vi "auto left.vi"() -> ()   [LabVIEW 2012, in "Omni2013.lvrbt"]
uses:
  Omni2013.lvrbt
  <vilib>/NXT/Hardware/Plugins/Tetrix 180 deg Servo/Tetrix180ServoAddress.ctl
  <vilib>/NXT/Hardware/Plugins/Tetrix DC Motor/TetrixDCMotorAddress.ctl
  <vilib>/NXT/Block Support/NXT_InputPort.ctl
  <vilib>/NXT/HiTechnic/HiTechnic Controls/HiTechnic Port.ctl
  <vilib>/NXT/Dual Mode Library/Waits/Wait_Num(msec).vi
  <vilib>/NXT/NXTIO Xnodes/NXTIONodeSubVIs/TETRIX IO Move Servos.vi
  <vilib>/NXT/NXTIO Xnodes/NXTIONodeSubVIs/TETRIX IO Move DC Motors.vi
  <vilib>/NXT/HiTechnic/HiTechnic Config/HiTechnic IRSeeker Mode1200Hz.vi
  <vilib>/NXT/Dual Mode Library/Sensors/Sonar_cm.vi
  <vilib>/NXT/Dual Mode Library/Display/drawNumber.vi
  <vilib>/NXT/HiTechnic/HiTechnic Read/HiTechnic IRSeeker Sensor_DC all.vi
  <vilib>/NXT/Dual Mode Library/Sensors/Light_On.vi
  <vilib>/NXT/NXTIO Xnodes/AddressXNode/NXTIOAddress.xnode
  <vilib>/NXT/NXTIO Xnodes/NXTIOXNode/NXTIO.xnode
  <vilib>/NXT/Subs/LVHSConnector.ctl
  <vilib>/NXT/LegoClasses/BrickReference/BrickReference.lvclass
panel:
  in  "Rotation":dbl
  in  "Translation L&R":dbl
  in  "Translation U&D":dbl
  in  "Initial Time":dbl
  out "Enabled":bool
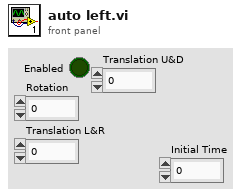
[diagram p1: front panel]
types:
  T1 = typedef "LVHSConnector.ctl" = refnum<class "BrickReference.lvclass">
  T2 = typedef "HiTechnic Port.ctl" = cluster{"Port":T3, "MUX Port":u8}
  T3 = typedef "NXT_InputPort.ctl" = u8
  T4 = typedef "TetrixDCMotorAddress.ctl" = i16
  T5 = cluster{"TetrixDCMotor":T4, "TetrixDCMotor 2":T4}
  T6 = typedef "Tetrix180ServoAddress.ctl" = i16
  T7 = cluster{"Direction (0-9)":i16, "Signal Strength (Array)":u8[]}
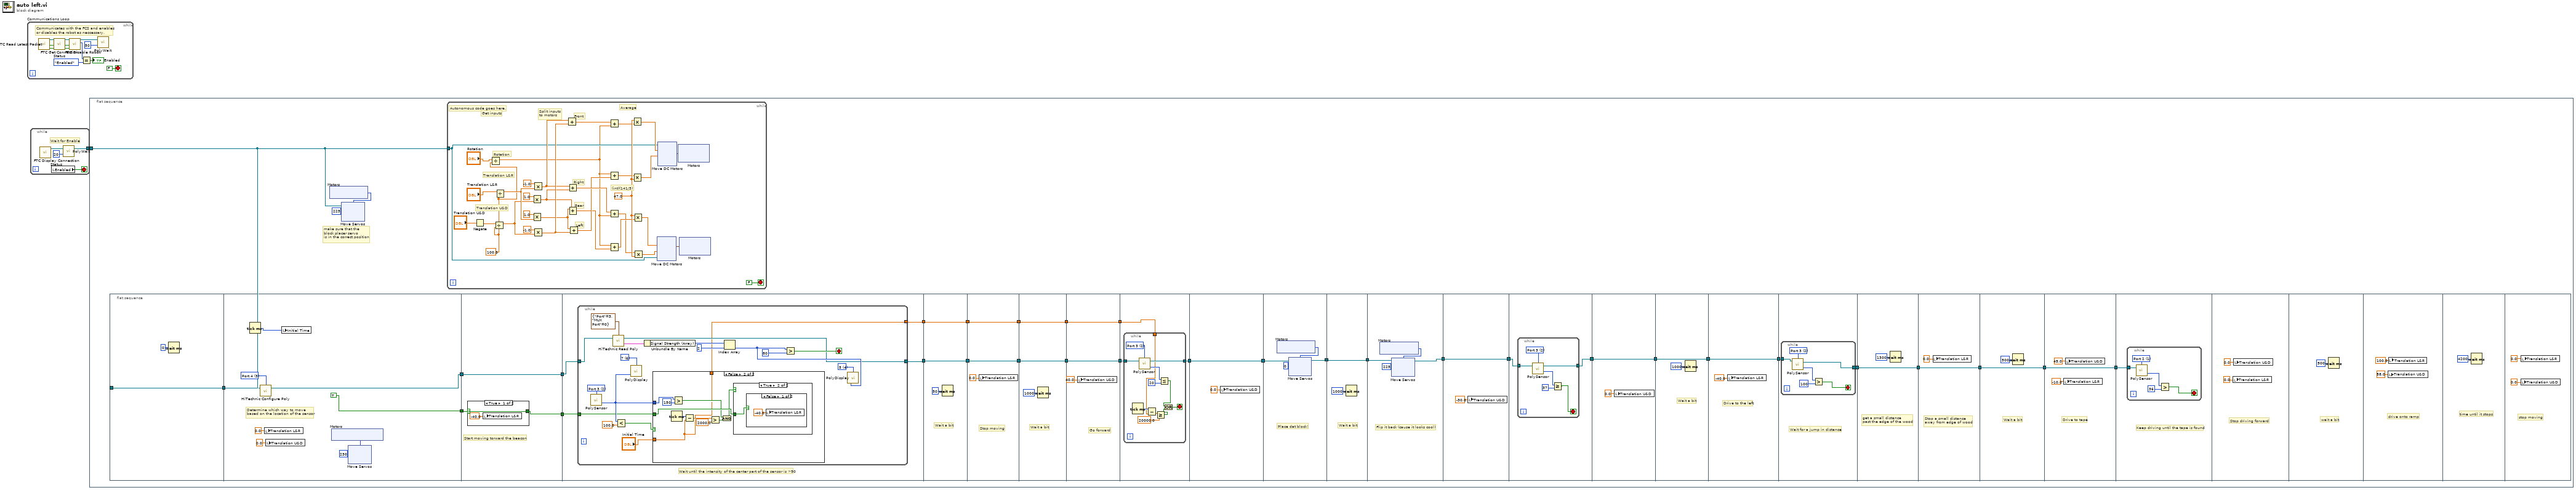
[diagram p0: block diagram]
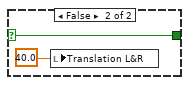
[diagram p2: hidden frame]
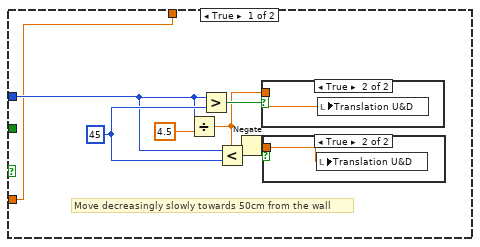
[diagram p3: hidden frame]
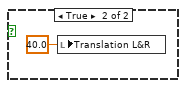
[diagram p7: hidden frame]
diagram:
  n1 = while "Communications Loop" {
    stop <- FALSE stop-if-true
    # "Communicates with the FCS and enables \nor disables the robot as neccessary."
    n2 = call <vilib>:"FTC Read Latest Packet.vi"() -> ("Packet Received?"=w11:bool, "Stopped?"=w10:bool, "NXT"=w13:T1)  [unwired: 6 in, 3 out]
    n3 = call <vilib>:"FTC Get Connection Status.vi"("Packet Received?"=w11, "Stopped?"=w10, "NXT"=w13) -> ("Online?"=w2:bool, "Stopped?"=w3:bool, "NXT"=w12:T1)  [unwired: 5 in]
    n4 = call <vilib>:"FTC Disable Robot.vi"("Online?"=w2, "Stopped?"=w3, "NXT"=w12) -> ("Enabled?"=w6:enum16{"Disabled", "Enabled"}, "NXT"=w8:T1)  [unwired: 3 in]
    n5 = Equal?(x=w6, y=enum16{"Disabled", "Enabled"}."Enabled") -> (x = y?=→"Enabled":bool)
    n6 = call-poly <vilib>:"PolyWait.vi"("Time (100 msec)"=u32 50 ("Time (msec)"), "NXT"=w8) -> ()  [unwired: 2 in, 1 out]
  }
  n7 = while {
    tunnel: [w15] -> w1
    stop <- w16 stop-if-true
    # "Wait for Enable"
    n8 = call <vilib>:"FTC Display Connection Status.vi"() -> ("NXT"=w14:T1)  [unwired: 11 in]
    n9 = local read "Enabled"() -> (w16:bool)
    n10 = call-poly <vilib>:"PolyWait.vi"("Time (100 msec)"=u32 20 ("Time (msec)"), "NXT"=w14) -> ("NXT"=w15:T1)  [unwired: 2 in]
  }
  n11 = flat-sequence {
    tunnel: w1 -> [w48]
    frame #0 {
      # "make sure that the \nblock placer servo \nis in the correct position"
      n12 = flat-sequence {
        tunnel: w48 -> [w60]
        tunnel: [w60] -> w29
        tunnel: [TRUE] -> w31
        tunnel: [w68] -> w30
        tunnel: w29 -> [w64]
        tunnel: [w80] -> w45
        tunnel: w31 -> [w79]
        tunnel: w30 -> [w80]
        tunnel: [w78] -> w39
        tunnel: w45 -> [w88]
        tunnel: [w87] -> w47
        tunnel: w39 -> [w86]
        tunnel: [w85] -> w18
        tunnel: w47 -> [w132]
        tunnel: [w132] -> w46
        tunnel: [w130] -> w19
        tunnel: w18 -> [w130]
        tunnel: [w134] -> w44
        tunnel: w46 -> [w134]
        tunnel: [w133] -> w20
        tunnel: w19 -> [w133]
        tunnel: [w138] -> w40
        tunnel: w44 -> [w138]
        tunnel: [w136] -> w21
        tunnel: w20 -> [w136]
        tunnel: w40 -> [w141]
        tunnel: [w141] -> w43
        tunnel: [w139] -> w22
        tunnel: w21 -> [w139]
        tunnel: w43 -> [w144]
        tunnel: [w143] -> w28
        tunnel: w22 -> [w142]
        tunnel: [w157] -> w27
        tunnel: w28 -> [w157]
        tunnel: w27 -> [w160]
        tunnel: [w159] -> w42
        tunnel: w42 -> [w172]
        tunnel: [w172] -> w41
        tunnel: w41 -> [w174]
        tunnel: [w173] -> w26
        tunnel: w26 -> [w186]
        tunnel: [w186] -> w25
        tunnel: w25 -> [w188]
        tunnel: [w187] -> w24
        tunnel: w24 -> [w196]
        tunnel: [w196] -> w23
        tunnel: [w197] -> w37
        tunnel: w23 -> [w197]
        tunnel: [w199] -> w38
        tunnel: w37 -> [w199]
        tunnel: w38 -> [w202]
        tunnel: [w201] -> w32
        tunnel: [w209] -> w33
        tunnel: w32 -> [w209]
        tunnel: [w211] -> w34
        tunnel: w33 -> [w211]
        tunnel: [w213] -> w35
        tunnel: w34 -> [w213]
        tunnel: [w215] -> w36
        tunnel: w35 -> [w215]
        tunnel: w36 -> [w218]
        frame #0 {
          n13 = Wait (ms)(milliseconds to wait=u32 0) -> ()  [unwired: 1 out]
        }
        frame #1 {
          w67 = T3 3 items=["Port 1", "Port 2", "Port 3", "Port 4"] ("Port")
          # "Determine which way to move \nbased on the location of the sensor"
          n14 = Tick Count (ms)() -> (millisecond timer value=w63:u32)
          n15 = call-poly <vilib>:"HiTechnic Configure Poly.vi"("NXT"=w64, "Port"=w67) -> ("NXT"=w68:T1)  [unwired: 2 in]
          n16 = local write "Translation L&R"(0.0 ("Translation L&R")) -> ()
          n17 = local write "Translation U&D"(0.0 ("Translation U&D")) -> ()
          n18 = local write "Initial Time"(w63) -> ()
          n19 = xnode "Motors"() -> ("Motor"=w62:T6)
          n20 = xnode "Move Servos"("Position 1"=u8 230, "Servos"=w62) -> ()  [unwired: 1 in, 1 out]
        }
        frame #2 {
          # "Start moving torward the beacon"
          n21 = case shown="True" w79 {
            selector: w79 -> [w81 w83]
            tunnel: [w81 w83] -> w78
            frame True {
              n22 = local write "Translation L&R"(-40.0 ("Translation L&R")) -> ()
            }
            frame False {
              n23 = local write "Translation L&R"(40.0 ("Translation L&R")) -> ()
            }
          }
        }
        frame #3 {
          # "Wait until the intensity of the center part of the sensor is >90"
          n24 = while {
            tunnel: w88 -> [w98]
            tunnel: [w96] -> w87
            tunnel: w86 -> [w91]
            tunnel: [w90] -> w85
            stop <- w102 stop-if-true
            w95 = i16 6 items=["1", "2", "3", "4", "5", "6", "7", "8"] ("Line")
            w97 = T3 2 items=["Port 1", "Port 2", "Port 3", "Port 4"] ("Port (Port 4)")
            w101 = i16 4 items=["1", "2", "3", "4", "5", "6", "7", "8"] ("Line")
            n25 = call-poly <vilib>:"PolySensor.vi"("Port (Port 4)"=w97) -> ("Distance (cm)"=w93:i16)  [unwired: 2 in, 1 out]
            n26 = call-poly <vilib>:"HiTechnic Read Poly.vi"("NXT"=w98, "Port/MUX"=T2 {"Port"=3, "MUX Port"=0}) -> ("All Info"=w105:T7, "NXT"=w96:T1)  [unwired: 1 in]
            n27 = Less?(x=w93, y=100.0) -> (x < y?=w92:bool)
            n28 = call-poly <vilib>:"PolyDisplay.vi"("number"=w93, "Line"=w95) -> ()  [unwired: 2 in, 1 out]
            n29 = Unbundle By Name(w105) -> ("Signal Strength (Array)"=w104:u8[])
            n30 = case shown="False" w92 {
              tunnel: w93 -> [w110 w126]
              tunnel: w91 -> [_ w124]
              tunnel: [w107 w117] -> w90
              tunnel: "Initial Time" -> [w107 w117]
              frame True {
                w112 = i16 45 ("y")
                # "Move decreasingly slowly towards 50cm from the wall"
                n31 = Divide(x=w110, y=4.5) -> (x/y=w109:dbl)
                n32 = Greater?(x=w110, y=w112) -> (0:w113:bool)
                n33 = Less?(x=w110, y=w112) -> (x < y?=w114:bool)
                n34 = Negate(x=w109) -> (-x=w108:dbl)
                n35 = case shown="True" w113 {
                  tunnel: w109 -> [_ w115]
                  frame False {
                  }
                  frame True {
                    n36 = local write "Translation U&D"(w115) -> ()
                  }
                }
                n37 = case shown="True" w114 {
                  tunnel: w108 -> [_ w116]
                  frame False {
                  }
                  frame True {
                    n38 = local write "Translation U&D"(w116) -> ()
                  }
                }
              }
              frame False {
                n39 = Tick Count (ms)() -> (millisecond timer value=w123:u32)
                n40 = Greater?(x=w126, y=i16 150) -> (0:w119:bool)
                n41 = Subtract(x=w123, y=w117) -> (x-y=w122:dbl)
                n42 = Greater?(x=w122, y=2000.0) -> (0:w118:bool)
                n43 = And(x=w119, y=w118) -> (x .and. y?=w120:bool)
                n44 = case shown="True" w120 {
                  tunnel: w124 -> [_ w127]
                  frame False {
                  }
                  frame True {
                    n45 = case shown="False" w127 {
                      frame False {
                        n46 = local write "Translation L&R"(-40.0 ("Translation L&R")) -> ()
                      }
                      frame True {
                        n47 = local write "Translation L&R"(40.0 ("Translation L&R")) -> ()
                      }
                    }
                  }
                }
              }
            }
            n48 = Index Array(array=w104, index=2) -> (element=w100:u8)
            n49 = Greater?(x=w100, y=u8 80) -> (0:w102:bool)
            n50 = call-poly <vilib>:"PolyDisplay.vi"("number"=w100, "Line"=w101) -> ()  [unwired: 2 in, 1 out]
          }
        }
        frame #4 {
          # "Wait a bit"
          n51 = Wait (ms)(milliseconds to wait=u32 50) -> ()  [unwired: 1 out]
        }
        frame #5 {
          # "Stop moving"
          n52 = local write "Translation L&R"(0.0 ("Translation L&R")) -> ()
        }
        frame #6 {
          # "Wait a bit"
          n53 = Wait (ms)(milliseconds to wait=u32 1000) -> ()  [unwired: 1 out]
        }
        frame #7 {
          # "Go forward"
          n54 = local write "Translation U&D"(40.0 ("Translation U&D")) -> ()
        }
        frame #8 {
          n55 = while {
            tunnel: w144 -> [w154]
            tunnel: [w153] -> w143
            tunnel: w142 -> [w150]
            stop <- w145 stop-if-true
            w152 = T3 2 items=["Port 1", "Port 2", "Port 3", "Port 4"] ("Port (Port 4)")
            n56 = Tick Count (ms)() -> (millisecond timer value=w151:u32)
            n57 = call-poly <vilib>:"PolySensor.vi"("NXT"=w154, "Port (Port 4)"=w152) -> ("Distance (cm)"=w156:i16, "NXT"=w153:T1)  [unwired: 1 in]
            n58 = Subtract(x=w151, y=w150) -> (x-y=w149:dbl)
            n59 = Greater Or Equal?(x=w149, y=20000.0) -> (x >= y?=w146:bool)
            n60 = Less Or Equal?(x=w156, y=i16 20) -> (x <= y?=w147:bool)
            n61 = Or(x=w147, y=w146) -> (x .or. y?=w145:bool)
          }
        }
        frame #9 {
          n62 = local write "Translation U&D"(0.0 ("Translation U&D")) -> ()
        }
        frame #10 {
          # "Place dat block!"
          n63 = xnode "Motors"() -> ("Motor"=w162:T6)
          n64 = xnode "Move Servos"("Position 1"=u8 0, "Servos"=w162, "NXT"=w160) -> ("NXT"=w159:T1)
        }
        frame #11 {
          # "Wait a bit"
          n65 = Wait (ms)(milliseconds to wait=u32 1000) -> ()  [unwired: 1 out]
        }
        frame #12 {
          # "Flip it back (cause it looks cool)"
          n66 = xnode "Motors"() -> ("Motor"=w176:T6)
          n67 = xnode "Move Servos"("Position 1"=u8 225, "Servos"=w176, "NXT"=w174) -> ("NXT"=w173:T1)
        }
        frame #13 {
          n68 = local write "Translation U&D"(-30.0 ("Translation U&D")) -> ()
        }
        frame #14 {
          n69 = while {
            tunnel: w188 -> [w194]
            tunnel: [w193] -> w187
            stop <- w191 stop-if-true
            w192 = T3 2 items=["Port 1", "Port 2", "Port 3", "Port 4"] ("Port (Port 4)")
            n70 = call-poly <vilib>:"PolySensor.vi"("NXT"=w194, "Port (Port 4)"=w192) -> ("Distance (cm)"=w190:i16, "NXT"=w193:T1)  [unwired: 1 in]
            n71 = Greater Or Equal?(x=w190, y=i16 37) -> (x >= y?=w191:bool)
          }
        }
        frame #15 {
          n72 = local write "Translation U&D"(0.0 ("Translation U&D")) -> ()
        }
        frame #16 {
          # "Wait a bit"
          n73 = Wait (ms)(milliseconds to wait=u32 1000) -> ()  [unwired: 1 out]
        }
        frame #17 {
          # "Drive to the left"
          n74 = local write "Translation L&R"(-40.0 ("Translation L&R")) -> ()
        }
        frame #18 {
          # "Wait for a jump in distance"
          n75 = while {
            tunnel: w202 -> [w204]
            tunnel: [w203] -> w201
            stop <- w206 stop-if-true
            w208 = T3 2 items=["Port 1", "Port 2", "Port 3", "Port 4"] ("Port (Port 4)")
            n76 = call-poly <vilib>:"PolySensor.vi"("NXT"=w204, "Port (Port 4)"=w208) -> ("Distance (cm)"=w205:i16, "NXT"=w203:T1)  [unwired: 1 in]
            n77 = Greater?(x=w205, y=i16 100) -> (0:w206:bool)
          }
        }
        frame #19 {
          # "get a small distance \npast the edge of the wood"
          n78 = Wait (ms)(milliseconds to wait=u32 1300) -> ()  [unwired: 1 out]
        }
        frame #20 {
          # "Stop a small distance \naway from edge of wood"
          n79 = local write "Translation L&R"(0.0 ("Translation L&R")) -> ()
        }
        frame #21 {
          # "Wait a bit"
          n80 = Wait (ms)(milliseconds to wait=u32 500) -> ()  [unwired: 1 out]
        }
        frame #22 {
          # "Drive to tape"
          n81 = local write "Translation L&R"(-10.0 ("Translation L&R")) -> ()
          n82 = local write "Translation U&D"(45.0 ("Translation U&D")) -> ()
        }
        frame #23 {
          # "Keep driving until the tape is found"
          n83 = while {
            tunnel: w218 -> [w219]
            stop <- w222 stop-if-true
            w221 = T3 1 items=["Port 1", "Port 2", "Port 3", "Port 4"] ("Port (Port 3)")
            n84 = call-poly <vilib>:"PolySensor.vi"("NXT"=w219, "Port (Port 3)"=w221) -> ("Scaled Value"=w220:i16)  [unwired: 1 in, 1 out]
            n85 = Greater?(x=w220, y=i16 36) -> (0:w222:bool)
          }
        }
        frame #24 {
          # "Stop driving forward"
          n86 = local write "Translation L&R"(0.0 ("Translation L&R")) -> ()
          n87 = local write "Translation U&D"(0.0 ("Translation U&D")) -> ()
        }
        frame #25 {
          # "wait a bit"
          n88 = Wait (ms)(milliseconds to wait=u32 500) -> ()  [unwired: 1 out]
        }
        frame #26 {
          # "drive onto ramp"
          n89 = local write "Translation U&D"(58.0 ("Translation U&D")) -> ()
          n90 = local write "Translation L&R"(100.0 ("Translation L&R")) -> ()
        }
        frame #27 {
          # "time until it stops"
          n91 = Wait (ms)(milliseconds to wait=u32 4200) -> ()  [unwired: 1 out]
        }
        frame #28 {
          # "stop moving"
          n92 = local write "Translation U&D"(0.0 ("Translation U&D")) -> ()
          n93 = local write "Translation L&R"(0.0 ("Translation L&R")) -> ()
        }
      }
      n94 = xnode "Motors"() -> ("Motor"=w50:T6)
      n95 = xnode "Move Servos"("Position 1"=u8 225, "Servos"=w50, "NXT"=w48) -> ()  [unwired: 1 out]
      n96 = while {
        tunnel: w48 -> [w237]
        stop <- FALSE stop-if-true
        w233 = 100.0 ("y")
        w264 = 47.0 ("y")
        # "Average"
        # "Left"
        # "Rear"
        # "Right"
        # "Front"
        # "(int)(141/3)"
        # "Split inputs to motors"
        # "Get inputs"
        # "Translation U&D"
        # "Rotation"
        # "Translation L&R"
        # "Autonomous code goes here."
        n97 = Negate(x="Translation U&D") -> (-x=w232:dbl)
        n98 = Divide(x="Rotation", y=w233) -> (x/y=w234:dbl)
        n99 = Divide(x=w232, y=w233) -> (x/y=w235:dbl)
        n100 = Divide(x="Translation L&R", y=w233) -> (x/y=w236:dbl)
        n101 = Multiply(x=1.0, y=w235) -> (x*y=w258:dbl)
        n102 = Multiply(x=1.0, y=w236) -> (x*y=w247:dbl)
        n103 = Multiply(x=-1.0, y=w236) -> (x*y=w246:dbl)
        n104 = Multiply(x=-1.0, y=w235) -> (x*y=w259:dbl)
        n105 = Add(x=w246, y=w259) -> (x+y=w243:dbl)
        n106 = Add(x=w246, y=w258) -> (x+y=w245:dbl)
        n107 = Add(x=w247, y=w258) -> (x+y=w242:dbl)
        n108 = Add(x=w247, y=w259) -> (x+y=w244:dbl)
        n109 = Add(x=w243, y=w234) -> (x+y=w262:dbl)
        n110 = Add(x=w234, y=w244) -> (x+y=w261:dbl)
        n111 = Add(x=w245, y=w234) -> (x+y=w260:dbl)
        n112 = Add(x=w234, y=w242) -> (x+y=w263:dbl)
        n113 = Multiply(x=w264, y=w262) -> (x*y=w253:dbl)
        n114 = Multiply(x=w261, y=w264) -> (x*y=w254:dbl)
        n115 = Multiply(x=w264, y=w263) -> (x*y=w257:dbl)
        n116 = Multiply(x=w260, y=w264) -> (x*y=w256:dbl)
        n117 = xnode "Motors"() -> ("Motor"=w252:cluster{"TetrixDCMotor":T4, "TetrixDCMotor":T4})
        n118 = xnode "Move DC Motors"("Power/Speed 2"=w254, "Power/Speed 1"=w253, "Motors"=w252, "NXT"=w237) -> ()  [unwired: 1 out]
        n119 = xnode "Motors"() -> ("Motor"=w255:cluster{"TetrixDCMotor":T4, "TetrixDCMotor":T4})
        n120 = xnode "Move DC Motors"("Power/Speed 2"=w256, "Power/Speed 1"=w257, "Motors"=w255, "NXT"=w237) -> ()  [unwired: 1 out]
      }
    }
  }
